vi "Channel_SetValues.vi"(7 "Data In":dbl[](array[numeric]), 8 "error in (no error)":errorcluster, 10 "Channel Count":u32, 11 "Channel in":refnum<class "Channel.lvclass">) -> (0 "error out":errorcluster, 2 "Channel Count Out":u32, 3 "Channel out":refnum<class "Channel.lvclass">)   [LabVIEW 2023, in "Channel.lvclass"]
doc: "Set the current channel value."
uses:
  Channel.lvclass
  Channel.lvclass/Channel.ctl
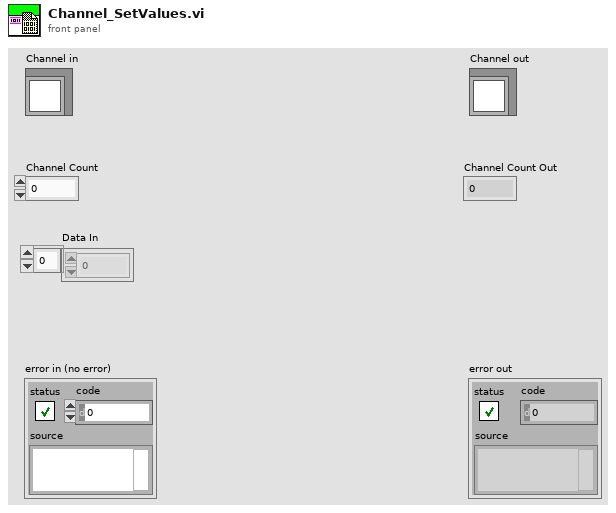
[diagram p1: front panel]
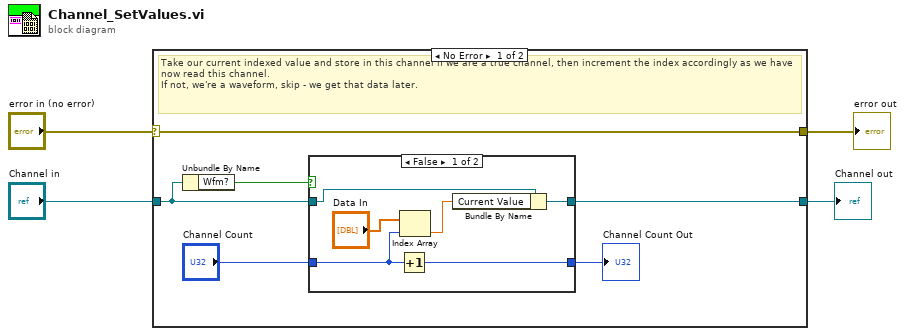
[diagram p0: block diagram]
diagram:
  n1 = case shown="No Error" "error in (no error)" {
    selector: "error in (no error)" -> [w10 w20]
    tunnel: [w10 w20] -> w3
    tunnel: [w5 w19] -> w1
    tunnel: "Channel in" -> [w6 w19]
    frame No Error {
      # "Take our current indexed value and store in this channel if we are a true channel, then increment the index accordingly as we have now read this channel.\nIf not, we're a waveform, skip - we get that data later."
      n2 = Unbundle By Name(w6) -> ("Wfm?"=w9:bool)
      n3 = case shown="False" w9 {
        tunnel: "Channel Count" -> [w12 w18]
        tunnel: [w16 w18] -> w7
        tunnel: w6 -> [w15 w17]
        tunnel: [w14 w17] -> w5
        frame False {
          n4 = Increment(x=w12) -> (x+1=w16:u32)
          n5 = Index Array(array="Data In", index=w12) -> (element=w11:dbl)
          n6 = Bundle By Name(cluster=w15, "Current Value"=w11) -> (w14:refnum<class "Channel.lvclass">)
        }
        frame True {
        }
      }
      "Channel Count Out" <- w7
    }
    frame Error {
    }
  }
  "error out" <- w3
  "Channel out" <- w1
